vi "DriveToPidRange.vi"(1 "Max Power":dbl) -> (0 "PID Range":T1)   [LabVIEW 2016]
uses:
  <userlib>/836-libraries/Drive/Drive_Code_V2/Drive_Code_Support/PidClusters/PidRange.ctl
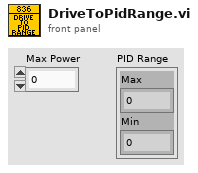
[diagram p1: front panel]
types:
  T1 = typedef "PidRange.ctl" = cluster{"Max":dbl, "Min":dbl}
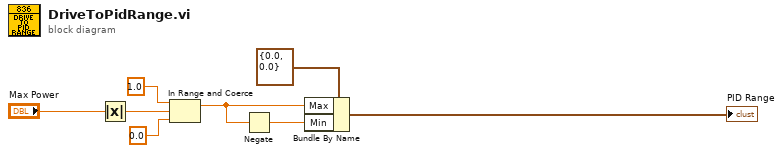
[diagram p0: block diagram]
diagram:
  n1 = Absolute Value(x="Max Power") -> (abs(x)=w5:dbl)
  n2 = In Range and Coerce(upper limit=1.0, x=w5, lower limit=0.0) -> (coerced(x)=w7:dbl)  [unwired: 1 out]
  n3 = Negate(x=w7) -> (-x=w8:dbl)
  n4 = Bundle By Name(cluster=T1 {"Max"=0.0, "Min"=0.0}, "Max"=w7, "Min"=w8) -> (→"PID Range":T1)
